vi "GenerateRuleList.vi"(8 "error in (no error)":errorcluster, 11 "CDependencyInspector in":refnum<class "CDependencyInspection.lvclass">) -> (0 "error out":errorcluster, 3 "CDependencyInspector out":refnum<class "CDependencyInspection.lvclass">)   [LabVIEW 2020, in "DependencyInspection.lvlib" / "CDependencyInspection.lvclass"]
uses:
  CDependencyInspection.lvclass
  CDependencyInspection.lvclass/CDependencyInspection.ctl
  obj/Addons/LabVIEWObjectInterfaces.lvlibp/ErrorManager/ErrorManager/ErrorType.ctl
  obj/Addons/ExtensionInterfaces.lvlibp/IRuleFileParser/IRuleFileParser.lvclass
  obj/Addons/ErrorManager.lvlibp/ErrorManager/ErrorManager.lvclass
  obj/Addons/LabVIEWObjectInterfaces.lvlibp/LabVIEWObjectInterfaces/IErrorManager/IErrorManager.lvclass
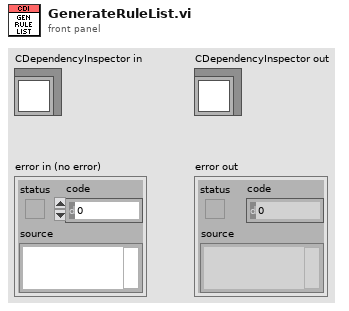
[diagram p1: front panel]
types:
  T1 = typedef "ExtensionInterfaces.lvlibp/IRuleFileParser.lvclass/RulesDefinition.ctl" = cluster{"Rule":cluster{"Delimited name":string, "Concession?":bool, "Layer":string}[]}[]
  T2 = typedef "LabVIEWObjectInterfaces.lvlibp/IErrorManager.lvclass/ErrorType.ctl" = enum16{"Info", "Warning", "Error"}
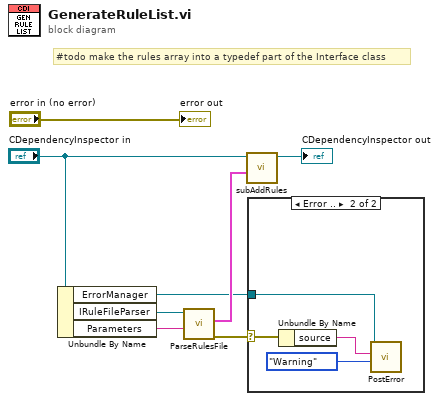
[diagram p0: block diagram]
diagram:
  # "#todo make the rules array into a typedef part of the Interface class"
  n1 = Unbundle By Name("CDependencyInspector in") -> ("ErrorManager"=w3:refnum<class "ErrorManager.lvclass">, "IRuleFileParser"=w6:refnum<class "IRuleFileParser.lvclass">, "Parameters"=w1:string)
  n2 = call-dynamic "ParseRulesFile.vi"("Parameters"=w1, "IRuleFileParser in"=w6) -> ("error out"=w4:errorcluster, "Rules"=w5:T1)  [unwired: 7 in, 1 out]
  n3 = call "subAddRules.vi"("Rules"=w5, "CDependencyInspector in"="CDependencyInspector in") -> ("CDependencyInspector out"=→"CDependencyInspector out":refnum<class "CDependencyInspection.lvclass">)  [unwired: 8 in, 1 out]
  n4 = case shown="Error .." w4 {
    selector: w4 -> [_ w10]
    tunnel: w3 -> [_ w11]
    frame No Error {
    }
    frame Error {
      n5 = Unbundle By Name(w10) -> ("source"=w9:string)
      n6 = call-dynamic "PostError.vi"("Type"=ErrorType."Warning", "Message"=w9, "ErrorManager in"=w11) -> ()  [unwired: 7 in, 2 out]
    }
  }
  "error out" <- "error in (no error)"
